vi "SwitchStates.vi"(8 "spitCube":bool, 9 "feedCube":bool, 10 "setSetpoint":bool) -> ()   [LabVIEW 2017]
uses:
  Implementation/Intake Operations.ctl
panel:
  out "number":u32
  # "input to the VI"
  # "output from the VI"
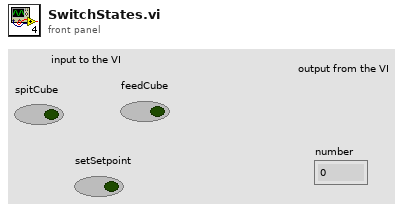
[diagram p1: front panel]
types:
  T1 = typedef "Intake Operations.ctl" = enum16{"Reserve", "Read Current", "Immediate", "idle", "setSetpoint", "feed", "spit"}
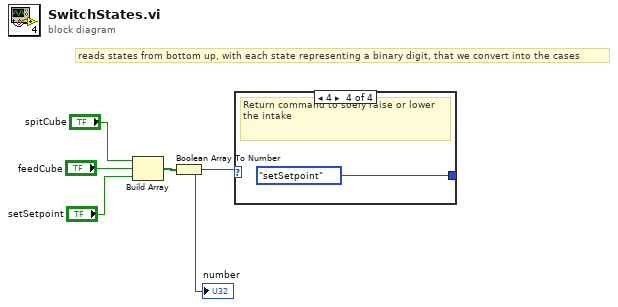
[diagram p0: block diagram]
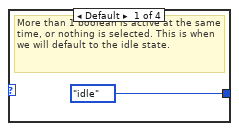
[diagram p2: hidden frame]
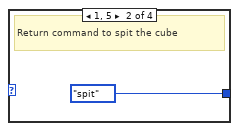
[diagram p3: hidden frame]
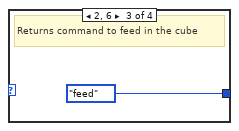
[diagram p4: hidden frame]
diagram:
  # "reads states from bottom up, with each state representing a binary digit, that we convert into the cases"
  n1 = Build Array("spitCube", "feedCube", "setSetpoint") -> (w4:bool[])
  n2 = Boolean Array To Number(Boolean array=w4) -> (number=w5:u32)
  "number" <- w5
  n3 = case shown="4" w5 {
    tunnel: [Intake_Operations."idle" ("Enum") Intake_Operations."spit" ("Enum") Intake_Operations."feed" ("Enum") Intake_Operations."setSetpoint" ("Enum")] -> _
    frame Default {
      # "More than 1 boolean is active at the same time, or nothing is selected. This is when we will default to the idle state."
    }
    frame 1, 5 {
      # "Return command to spit the cube"
    }
    frame 2, 6 {
      # "Returns command to feed in the cube"
    }
    frame 4 {
      # "Return command to soely raise or lower the intake"
    }
  }
